vi "Read Process SV.vi"(8 "error in (no error)":errorcluster, 11 "EMKO in":refnum<class "ESM-xx50.lvclass">) -> (0 "error out":errorcluster, 2 "Process SV":dbl format="%.2f", 3 "EMKO out":refnum<class "ESM-xx50.lvclass">)   [LabVIEW 2023, in "EMKO.lvlib" / "ESM-xx50.lvclass"]
uses:
  ESM-xx50.lvclass
  ESM-xx50.lvclass/ESM-xx50.ctl
  <vilib>/Modbus/master/Modbus Master.lvclass
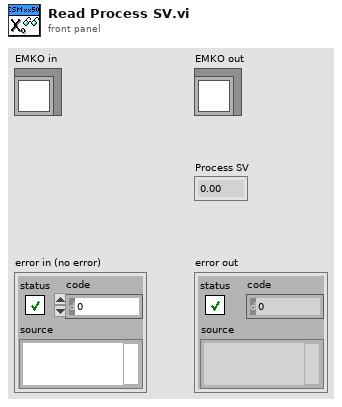
[diagram p1: front panel]
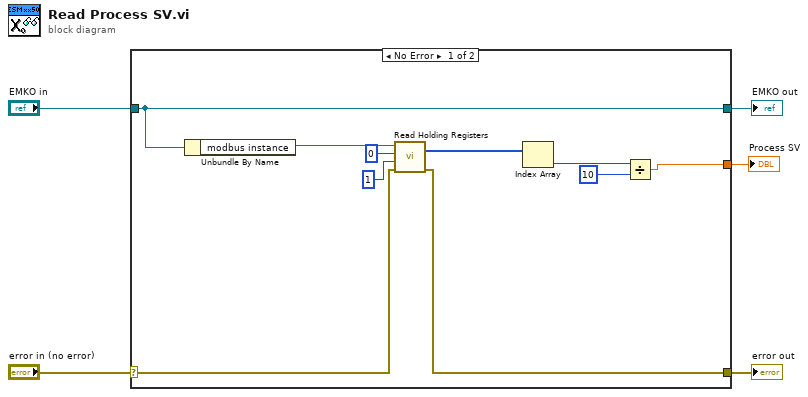
[diagram p0: block diagram]
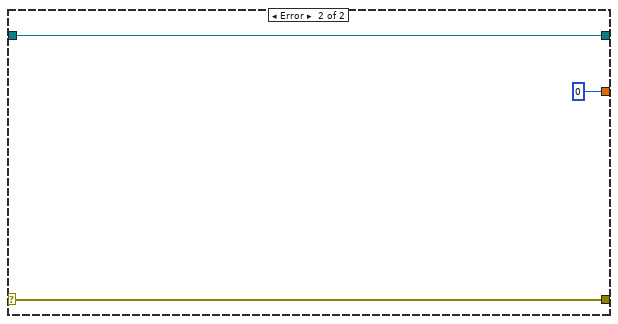
[diagram p2: hidden frame]
diagram:
  n1 = case shown="No Error" "error in (no error)" {
    selector: "error in (no error)" -> [w11 w18]
    tunnel: [w10 w18] -> w4
    tunnel: [w15 w17] -> w2
    tunnel: "EMKO in" -> [w15 w17]
    tunnel: [w7 u16 0 ("register")] -> w1
    frame No Error {
      n2 = Unbundle By Name(w15) -> ("modbus instance"=w14:refnum<class "Modbus Master.lvclass">)
      n3 = call-dynamic "Read Holding Registers.vi"("error in (no error)"=w11, "number of holding registers"=u16 1, "starting address"=u16 0, "Modbus master in"=w14) -> ("error out"=w10:errorcluster, "register values"=w9:u16[])  [unwired: 5 in, 1 out]
      n4 = Index Array(array=w9) -> (element=w8:u16)  [unwired: 1 in]
      n5 = Divide(x=w8, y=u16 10) -> (x/y=w7:dbl)
    }
    frame Error {
    }
  }
  "error out" <- w4
  "EMKO out" <- w2
  "Process SV" <- w1
